vi "DAQ-AO初始化(Sub VI).vi"(6 "output terminal configuration":i32(ring)=10083 items=["Default"=-1, "RSE"=10083, "Differential"=10106, "Pseudodifferential"=12529], 7 "sample mode":i32(ring)=10123 items=["Finite Samples"=10178, "Continuous Samples"=10123, "Hardware Timed Single Point"=12522], 8 "error in":errorcluster, 9 "minimum value":dbl=-2.0, 10 "maximum value":dbl=2.0, 11 "取樣頻率(Hz)":dbl=1000.0) -> (0 "error out":errorcluster, 3 "task out":refnum<k21>)   [LabVIEW 2010]
uses:
  <vilib>/DAQmx/create/channels.llb/DAQmx Create Channel (AO-Voltage-Basic).vi
  <vilib>/DAQmx/configure/timing.llb/DAQmx Timing (Sample Clock).vi
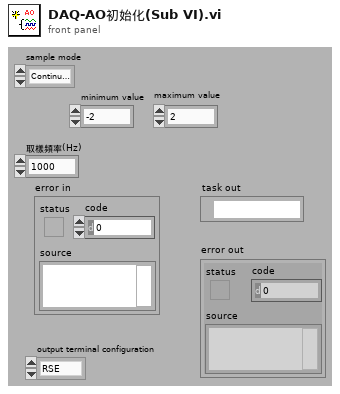
[diagram p1: front panel]
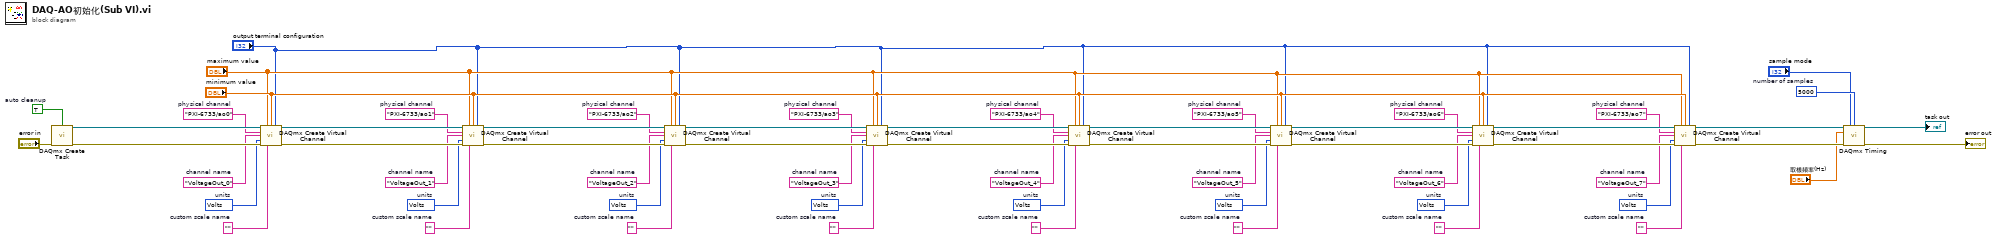
[diagram p0: block diagram]
diagram:
  w7 = 5000  # number of samples
  w10 = 10348 items=["Volts"=10348, "From Custom Scale"=10065]  # units
  w11 = "VoltageOut_7"  # channel name
  w13 = ""  # custom scale name
  w14 = "PXI-6733/ao7"  # physical channel
  w16 = 10348 items=["Volts"=10348, "From Custom Scale"=10065]  # units
  w17 = "VoltageOut_6"  # channel name
  w19 = ""  # custom scale name
  w20 = "PXI-6733/ao6"  # physical channel
  w22 = 10348 items=["Volts"=10348, "From Custom Scale"=10065]  # units
  w23 = "VoltageOut_5"  # channel name
  w25 = ""  # custom scale name
  w26 = "PXI-6733/ao5"  # physical channel
  w28 = 10348 items=["Volts"=10348, "From Custom Scale"=10065]  # units
  w29 = "VoltageOut_4"  # channel name
  w31 = ""  # custom scale name
  w32 = "PXI-6733/ao4"  # physical channel
  w34 = 10348 items=["Volts"=10348, "From Custom Scale"=10065]  # units
  w35 = "VoltageOut_3"  # channel name
  w37 = ""  # custom scale name
  w38 = "PXI-6733/ao3"  # physical channel
  w40 = 10348 items=["Volts"=10348, "From Custom Scale"=10065]  # units
  w41 = "VoltageOut_2"  # channel name
  w43 = ""  # custom scale name
  w44 = "PXI-6733/ao2"  # physical channel
  w46 = 10348 items=["Volts"=10348, "From Custom Scale"=10065]  # units
  w47 = "VoltageOut_1"  # channel name
  w49 = ""  # custom scale name
  w50 = "PXI-6733/ao1"  # physical channel
  w52 = 10348 items=["Volts"=10348, "From Custom Scale"=10065]  # units
  w53 = "VoltageOut_0"  # channel name
  w55 = ""  # custom scale name
  w56 = "PXI-6733/ao0"  # physical channel
  w58 = TRUE  # auto cleanup
  n1 = call <vilib>:"DAQmx Create Task.vi"("auto cleanup"=w58, "error in"="error in") -> ("task out"=w57:refnum<k21>, "error out"=w59:errorcluster)  [unwired: 12 in]
  n2 = call-poly <vilib>:"DAQmx Create Virtual Channel.vi"("task in"=w57, "maximum value"="maximum value", "minimum value"="minimum value", "output terminal configuration"="output terminal configuration", "physical channels"=w56, "name to assign"=w53, "units"=w52, "error in"=w59, "custom scale name"=w55) -> ("task out"=w51:refnum<k21>, "error out"=w54:errorcluster)  [unwired: 5 in]
  n3 = call-poly <vilib>:"DAQmx Create Virtual Channel.vi"("task in"=w51, "maximum value"="maximum value", "minimum value"="minimum value", "output terminal configuration"="output terminal configuration", "physical channels"=w50, "name to assign"=w47, "units"=w46, "error in"=w54, "custom scale name"=w49) -> ("task out"=w45:refnum<k21>, "error out"=w48:errorcluster)  [unwired: 5 in]
  n4 = call-poly <vilib>:"DAQmx Create Virtual Channel.vi"("task in"=w45, "maximum value"="maximum value", "minimum value"="minimum value", "output terminal configuration"="output terminal configuration", "physical channels"=w44, "name to assign"=w41, "units"=w40, "error in"=w48, "custom scale name"=w43) -> ("task out"=w39:refnum<k21>, "error out"=w42:errorcluster)  [unwired: 5 in]
  n5 = call-poly <vilib>:"DAQmx Create Virtual Channel.vi"("task in"=w39, "maximum value"="maximum value", "minimum value"="minimum value", "output terminal configuration"="output terminal configuration", "physical channels"=w38, "name to assign"=w35, "units"=w34, "error in"=w42, "custom scale name"=w37) -> ("task out"=w33:refnum<k21>, "error out"=w36:errorcluster)  [unwired: 5 in]
  n6 = call-poly <vilib>:"DAQmx Create Virtual Channel.vi"("task in"=w33, "maximum value"="maximum value", "minimum value"="minimum value", "output terminal configuration"="output terminal configuration", "physical channels"=w32, "name to assign"=w29, "units"=w28, "error in"=w36, "custom scale name"=w31) -> ("task out"=w27:refnum<k21>, "error out"=w30:errorcluster)  [unwired: 5 in]
  n7 = call-poly <vilib>:"DAQmx Create Virtual Channel.vi"("task in"=w27, "maximum value"="maximum value", "minimum value"="minimum value", "output terminal configuration"="output terminal configuration", "physical channels"=w26, "name to assign"=w23, "units"=w22, "error in"=w30, "custom scale name"=w25) -> ("task out"=w21:refnum<k21>, "error out"=w24:errorcluster)  [unwired: 5 in]
  n8 = call-poly <vilib>:"DAQmx Create Virtual Channel.vi"("task in"=w21, "maximum value"="maximum value", "minimum value"="minimum value", "output terminal configuration"="output terminal configuration", "physical channels"=w20, "name to assign"=w17, "units"=w16, "error in"=w24, "custom scale name"=w19) -> ("task out"=w15:refnum<k21>, "error out"=w18:errorcluster)  [unwired: 5 in]
  n9 = call-poly <vilib>:"DAQmx Create Virtual Channel.vi"("task in"=w15, "maximum value"="maximum value", "minimum value"="minimum value", "output terminal configuration"="output terminal configuration", "physical channels"=w14, "name to assign"=w11, "units"=w10, "error in"=w18, "custom scale name"=w13) -> ("task out"=w9:refnum<k21>, "error out"=w12:errorcluster)  [unwired: 5 in]
  n10 = call-poly <vilib>:"DAQmx Timing.vi"("task/channels in"=w9, "sample mode"="sample mode", "samples per channel"=w7, "rate"="取樣頻率(Hz)", "error in"=w12) -> ("task out"=→"task out":refnum<k21>, "error out"=→"error out":errorcluster)  [unwired: 9 in]
